vi "find_read_width.vi"(10 "timetags":u32[][](array[numeric]), 11 "T1_parameters":T1) -> (2 "mse":cluster{"read_widths_us":dbl[], "mse":dbl[]}, 3 "proposed_read_width_us":dbl)   [LabVIEW 2018]
uses:
  <vilib>/Analysis/1siggen.llb/Ramp Pattern by Delta.vi
  <vilib>/Analysis/NI_AALBase.lvlib
panel:
  in  "step_size_us":dbl=0.01
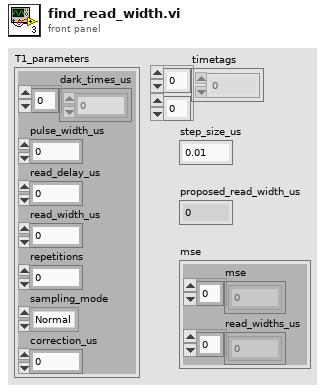
[diagram p1: front panel]
types:
  T1 = cluster{"dark_times_us":dbl[], "pulse_width_us":dbl, "read_delay_us":dbl, "read_width_us":dbl, "repetitions":i32, "sampling_mode":enum16{"Normal", "Sweep"}, "correction_us":dbl}
  T2 = cluster{"Ie":dbl, "Cm":dbl, "Tm":dbl, "C1":dbl, "T1":dbl, "mse":dbl}
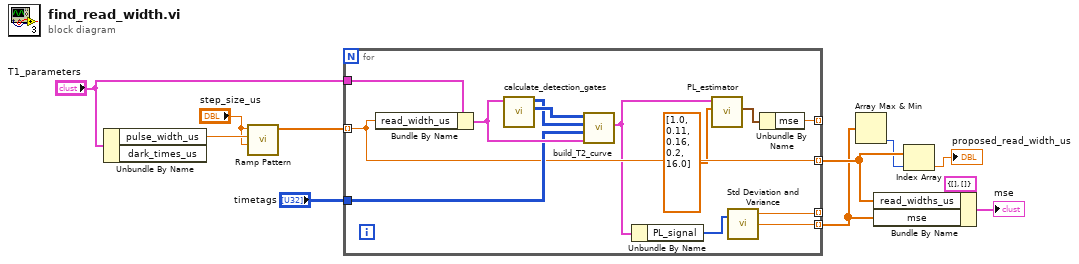
[diagram p0: block diagram]
diagram:
  n1 = Unbundle By Name("T1_parameters") -> ("pulse_width_us"=w11:dbl)  [unwired: 1 out]
  n2 = call-poly <vilib>:"Ramp Pattern.vi"("start"="step_size_us", "end"=w11, "delta"="step_size_us") -> ("Ramp Pattern"=w10:dbl[])  [unwired: 6 in, 2 out]
  n3 = for {
    tunnel: w10 -> [w19] mode=indexing
    tunnel: "T1_parameters" -> [w21]
    tunnel: "timetags" -> [w20]
    tunnel: [w19] -> w5 mode=indexing
    tunnel: [w16] -> _ mode=indexing
    tunnel: [w13] -> _ mode=indexing
    tunnel: [w12] -> w1 mode=indexing
    n4 = Bundle By Name(cluster=w21, "read_width_us"=w19) -> (w24:T1)
    n5 = call "calculate_detection_gates.vi"("T1_parameters"=w24) -> ("start_read"=w23:u32[][], "stop_read"=w22:u32[][])  [unwired: 9 in]
    n6 = call "build_T2_curve.vi"("T1_parameters"=w24, "timetags"=w20, "stop_read"=w22, "start_read"=w23) -> ("T1 curve"=w15:cluster{"dark_time_us":dbl[], "PL_signal":i32[]})  [unwired: 5 in, 2 out]
    n7 = Unbundle By Name(w15) -> ("PL_signal"=w14:i32[])
    n8 = call "PL_estimator.vi"("initial parameters"=dbl[] [1.0, 0.11, 0.16, 0.2, 16.0], "measured_signal"=w15) -> ("fit_parameters"=w17:T2)  [unwired: 7 in, 2 out]
    n9 = call <vilib>:"Std Deviation and Variance.vi"("X"=w14) -> ("mean"=w13:dbl, "standard deviation"=w12:dbl)  [unwired: 1 in, 1 out]
    n10 = Unbundle By Name(w17) -> ("mse"=w16:dbl)
  }
  n11 = Array Max & Min(array=w1) -> (min index (indices)=w2:i32)  [unwired: 3 out]
  n12 = Bundle By Name(cluster=cluster{"read_widths_us":dbl[], "mse":dbl[]} {"read_widths_us"=[], "mse"=[]} ("hist1-read_width"), "read_widths_us"=w5, "mse"=w1) -> (→"mse":cluster{"read_widths_us":dbl[], "mse":dbl[]})
  n13 = Index Array(array=w5, index=w2) -> (element=→"proposed_read_width_us":dbl)
